vi "picoamp_right.vi"() -> ()   [LabVIEW 2015]
uses:
  global_qaqc.vi
panel:
  out "Acquisition Frequency":string="1"
  out "Board Name":string
  in  "Open DataBase":bool
  out "Output file path":path
  out "?":bool
  in  "Stop":bool
  out "Results Chart":dbl(graph)
  out "Voltage value":string
  in  "Start Test":bool
  out "Measure time (s)":string="300"
  # "Picoammeter test"
  # "Passed"
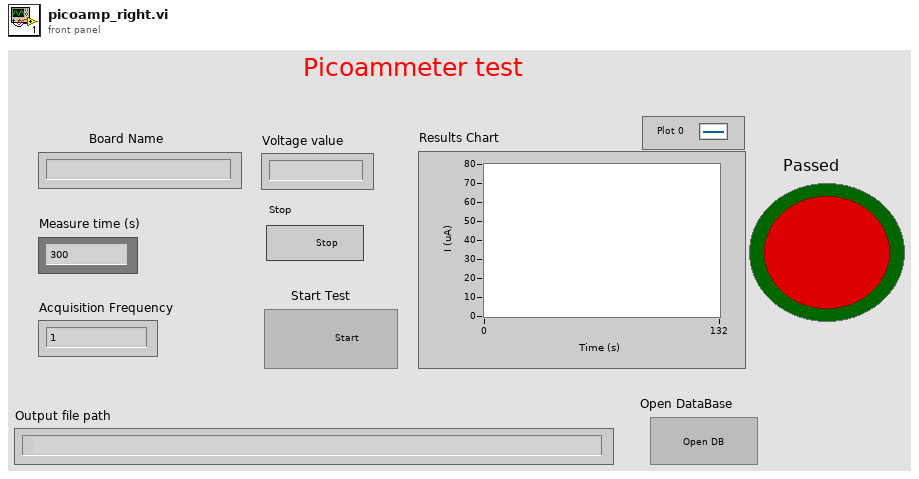
[diagram p1: front panel]
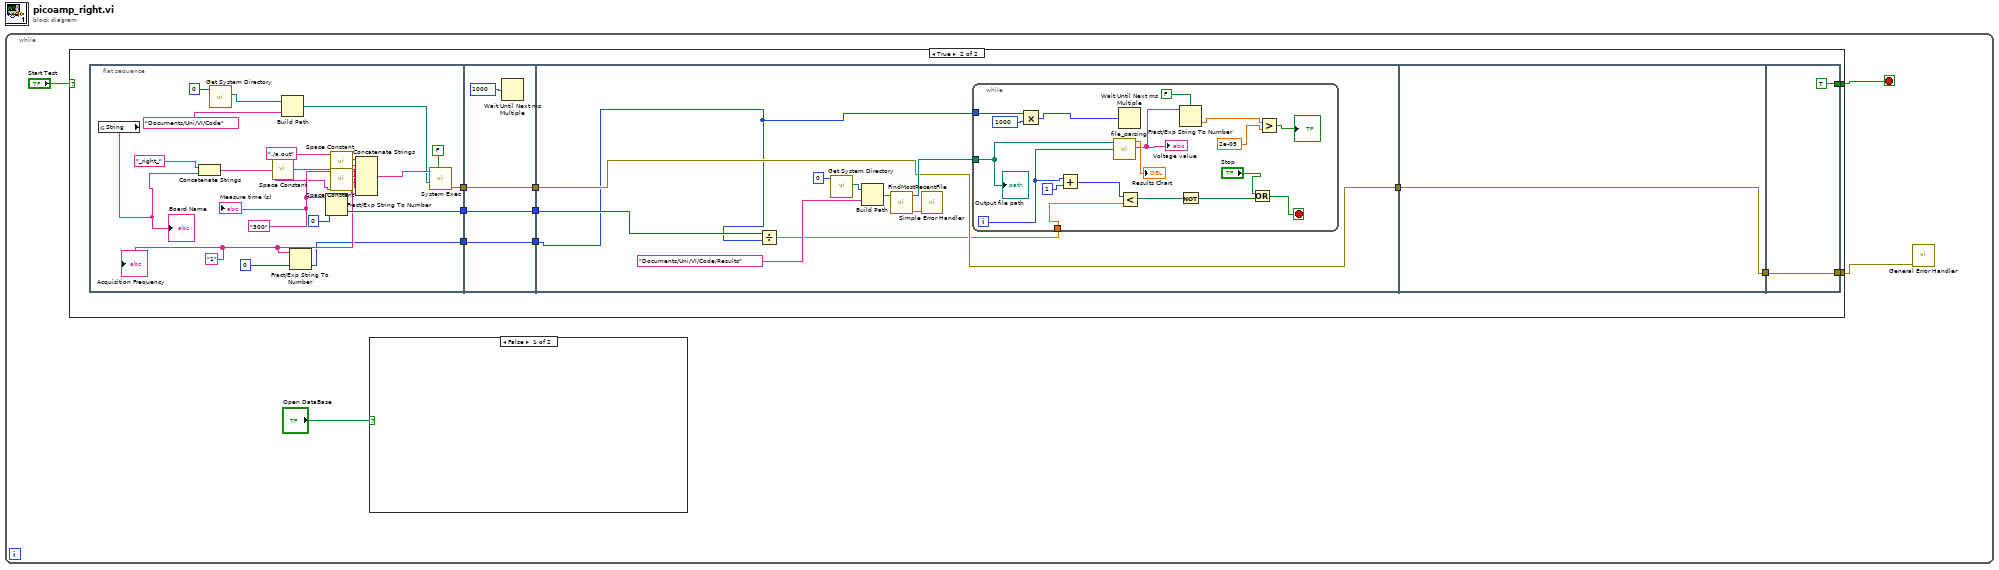
[diagram p0: block diagram]
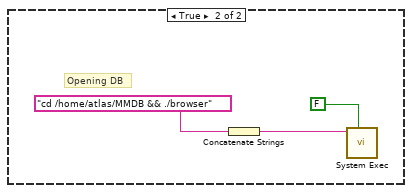
[diagram p2: hidden frame]
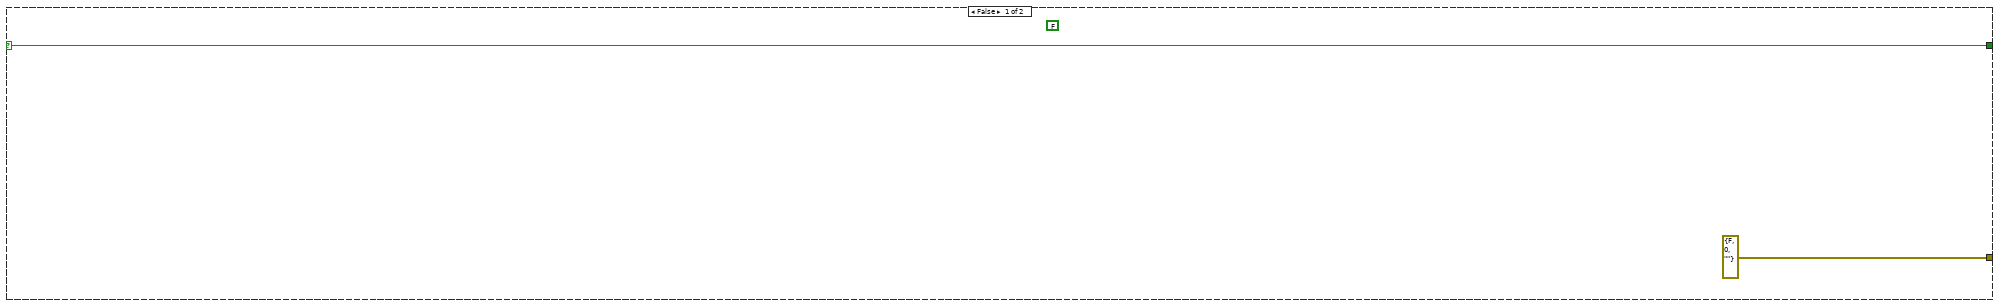
[diagram p3: hidden frame]
diagram:
  n1 = while {
    stop <- w3 stop-if-true
    n2 = case shown="True" "Start Test" {
      selector: "Start Test" -> [w9 _]
      tunnel: [w9 w19] -> w3
      tunnel: [errorcluster {"status"=FALSE, "code"=0, "source"=""} ("error out") w17] -> w2
      frame False {
        (unwired) FALSE
      }
      frame True {
        n3 = flat-sequence {
          tunnel: [w39] -> w16
          tunnel: [w24] -> w14
          tunnel: [w33] -> w12
          tunnel: w16 -> [w43]
          tunnel: [w43] -> w18
          tunnel: [w41] -> w15
          tunnel: w14 -> [w41]
          tunnel: [w40] -> w13
          tunnel: w12 -> [w40]
          tunnel: w18 -> [w47]
          tunnel: w15 -> [w45]
          tunnel: w13 -> [w46]
          tunnel: [w47] -> w11
          tunnel: w11 -> [w72]
          tunnel: [w72] -> w10
          tunnel: [TRUE] -> w19
          tunnel: [w73] -> w17
          tunnel: w10 -> [w73]
          frame #0 {
            w23 = "300" ("Measure time (s)")
            w25 = "1"
            n4 = global read "global_qaqc.vi" "String"() -> (w21:string)
            "Board Name" <- w21
            n5 = Concatenate Strings("_right_", w21) -> (w20:string)
            n6 = call <vilib>:"Get System Directory.vi"("system directory type"=0) -> ("system directory"=w29:path)  [unwired: 10 in]
            n7 = call <vilib>:"Space Constant.vi"() -> ("String"=w27:string)
            n8 = Build Path(base path=w29, name or relative path="Documents/Uni/VI/Code") -> (appended path=w28:path)
            n9 = Fract/Exp String To Number(string=w25, default (0 dbl)=0) -> (number=w24:i32)  [unwired: 2 in, 1 out]
            n10 = Fract/Exp String To Number(string=w23, default (0 dbl)=0) -> (number=w33:i32)  [unwired: 2 in, 1 out]
            n11 = call <vilib>:"Space Constant.vi"() -> ("String"=w37:string)
            n12 = call <vilib>:"Space Constant.vi"() -> ("String"=w38:string)
            n13 = Concatenate Strings("./a.out" ("String"), w37, w23, w38, w25, w27, w20) -> (w35:string)
            n14 = call <vilib>:"System Exec.vi"("wait until completion? (T)"=FALSE, "working directory"=w28, "command line"=w35) -> ("error out"=w39:errorcluster)  [unwired: 5 in, 3 out]
            "Measure time (s)" <- w23
            "Acquisition Frequency" <- w25
          }
          frame #1 {
            n15 = Wait Until Next ms Multiple(millisecond multiple=u32 1000) -> ()  [unwired: 1 out]
          }
          frame #2 {
            n16 = Divide(x=w46, y=w45) -> (x/y=w44:dbl)
            n17 = call <vilib>:"Get System Directory.vi"("system directory type"=0) -> ("system directory"=w51:path)  [unwired: 10 in]
            n18 = Build Path(base path=w51, name or relative path="Documents/Uni/VI/Code/Results") -> (appended path=w49:path)
            n19 = call "FindMostRecentFile.vi"("Folder Path In"=w49) -> ("error out"=w48:errorcluster, "File Path Out"=w53:path)  [unwired: 9 in]
            n20 = call <vilib>:"Simple Error Handler.vi"("error in (no error)"=w48) -> ()  [unwired: 4 in, 5 out]
            n21 = while {
              tunnel: w53 -> [w69]
              tunnel: w44 -> [w68]
              tunnel: w45 -> [w62]
              i -> [w64]
              stop <- w65 stop-if-true
              n22 = Multiply(x=w62, y=1000) -> (x*y=w56:i32)
              n23 = Add(x=w64, y=1) -> (x+y=w55:i32)
              n24 = call "file_parsing.vi"("File Path Control"=w69, "line index"=w64) -> ("Waveform Chart"=→"Results Chart":dbl, "String"=w61:string)  [unwired: 1 in, 2 out]
              "Voltage value" <- w61
              n25 = Wait Until Next ms Multiple(millisecond multiple=w56) -> ()  [unwired: 1 out]
              n26 = Less?(x=w55, y=w68) -> (x < y?=w67:bool)
              n27 = Fract/Exp String To Number(use system decimal point (T)=FALSE, string=w61) -> (number=w59:dbl)  [unwired: 2 in, 1 out]
              n28 = Not(x=w67) -> (.not. x?=w66:bool)
              n29 = Or(x="Stop", y=w66) -> (x .or. y?=w65:bool)
              n30 = Greater?(x=w59, y=2e-05) -> (0:→"?":bool)
              "Output file path" <- w69
            }
          }
          frame #3 {
          }
          frame #4 {
          }
        }
      }
    }
    n31 = case shown="False" "Open DataBase" {
      frame False {
      }
      frame True {
        # "Opening DB"
        n32 = Concatenate Strings("cd /home/atlas/MMDB && ./browser") -> (w6:string)
        n33 = call <vilib>:"System Exec.vi"("wait until completion? (T)"=FALSE, "command line"=w6) -> ()  [unwired: 6 in, 4 out]
      }
    }
    n34 = call <vilib>:"General Error Handler.vi"("error in (no error)"=w2) -> ()  [unwired: 10 in, 5 out]
  }
